vi "Temp Chamber Testing Log w subVIs ver 2.vi"() -> ()   [LabVIEW 2010]
uses:
  <vilib>/Analysis/Matrix/Datatypes/RealMatrix.ctl
  <vilib>/Utility/NIReport.llb/NI_report.lvclass
  <vilib>/Utility/NIReport.llb/Append Numeric Table to Report (wrap).vi
  <vilib>/Utility/NIReport.llb/Excel/NI_Excel.lvclass
  <vilib>/Analysis/Matrix/NI_Matrix.lvlib
panel:
  in  "Wait time (row 1) [mins] and iterations for that time (row 2)":T1
  out "error out":errorcluster
  in  "error in (no error)":errorcluster
  in  "Fiber Len (m)":dbl
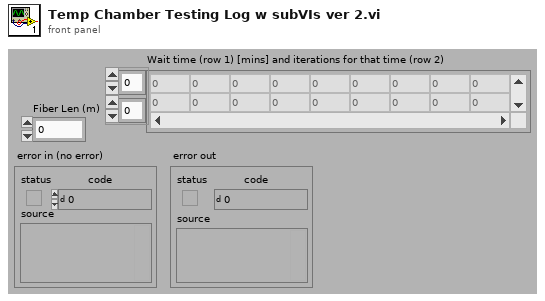
[diagram p1: front panel]
types:
  T1 = typedef "NI_Matrix.lvlib/RealMatrix.ctl" = dbl[][]
  T2 = enum16{"Standard Report", "HTML", "Word", "Excel"}
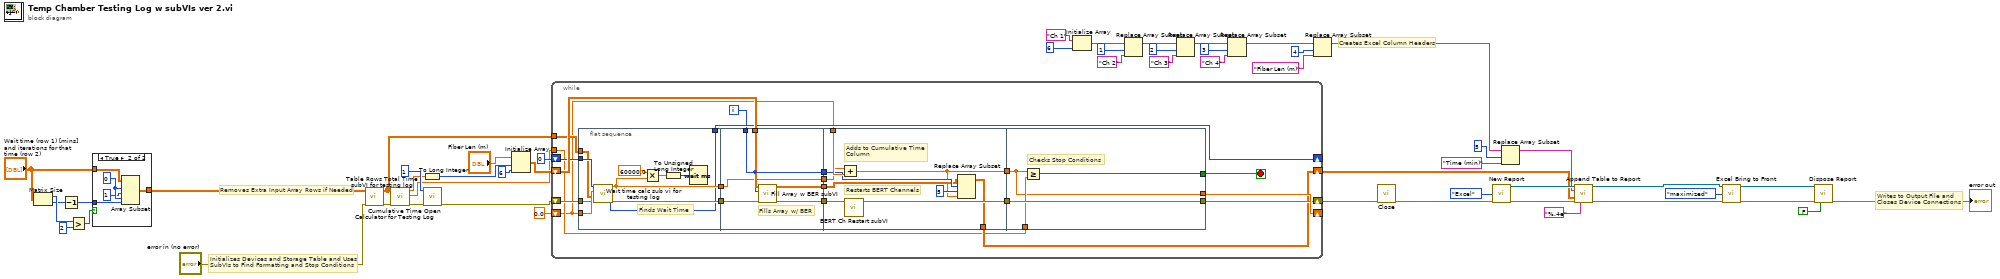
[diagram p0: block diagram]
diagram:
  # "Creates Excel Column Headers"
  # "Removes Extra Input Array Rows if Needed"
  # "Writes to Output File and \nCloses Device Connections"
  # "Initializes Devices and Storage Table and Uses\nSubVIs to Find Formatting and Stop Conditions"
  n1 = Matrix Size(0:"Wait time (row 1) [mins] and iterations for that time (row 2)") -> (1:w26:i32, 2:w22:i32)
  n2 = Decrement(x=w22) -> (x-1=w21:i32)
  n3 = Greater?(x=w26, y=2) -> (0:w24:bool)
  n4 = case shown="True" w24 {
    tunnel: "Wait time (row 1) [mins] and iterations for that time (row 2)" -> [w54 w59]
    tunnel: [w54 w58] -> w20
    tunnel: w21 -> [_ w55]
    frame False {
    }
    frame True {
      w57 = 0
      n5 = Array Subset(array=w59, index (row)=w57, length (row)=1, index (col)=w57, length (col)=w55) -> (w58:T1)
    }
  }
  n6 = call "Cumulative Time Calculator for Testing Log.vi"("error in (no error)"="error in (no error)", "Input Matrix"=w20) -> ("error out"=w27:errorcluster, "Output Matrix"=w29:T1)  [unwired: 8 in]
  n7 = call "Table Rows Total Time subVI for testing log.vi"("error in (no error)"=w27, "Input Matrix"=w29) -> ("error out"=w33:errorcluster, "Total Time (mins)"=w30:dbl, "# of Table Rows"=w32:dbl)  [unwired: 7 in]
  n8 = To Long Integer(number=w32) -> (32bit integer=w31:i32)
  n9 = call <instrlib>:"Open.vi"("error in (no error)"=w33, "type"=1) -> ("error out"=w50:errorcluster)  [unwired: 8 in, 1 out]
  n10 = Initialize Array("Fiber Len (m)", w31, 6) -> (w51:dbl[][])
  n11 = while {
    shift-right: [w65] -> w38
    shift-left: w51 -> [w79]
    shift-right: [w70] -> w35
    shift-left: w50 -> [w77]
    shift-right: [w75] -> _
    shift-left: 0.0 -> [w62]
    shift-right: [w73] -> _
    shift-left: 0 -> [w74]
    tunnel: w29 -> [w64]
    tunnel: w30 -> [w63]
    i -> [w71]
    stop <- w67 stop-if-true
    n12 = flat-sequence {
      tunnel: w77 -> [w86]
      tunnel: [w85] -> w76
      tunnel: w62 -> [w89]
      tunnel: w74 -> [w88]
      tunnel: [w84] -> w73
      tunnel: [w87] -> w72
      tunnel: w64 -> [w83]
      tunnel: w79 -> [w95]
      tunnel: w71 -> [w90]
      tunnel: [w91] -> w78
      tunnel: w76 -> [w92]
      tunnel: w72 -> [w93]
      tunnel: [w94] -> w66
      tunnel: [w93] -> w61
      tunnel: [w90] -> w60
      tunnel: w78 -> [w103]
      tunnel: w62 -> [w104]
      tunnel: [w96] -> w69
      tunnel: [w102] -> w68
      tunnel: w66 -> [w98]
      tunnel: [w97] -> w65
      tunnel: w61 -> [w101]
      tunnel: w60 -> [w99]
      tunnel: [w108] -> w70
      tunnel: [w105] -> w75
      tunnel: w69 -> [w105]
      tunnel: w68 -> [w108]
      tunnel: [w107] -> w67
      tunnel: w63 -> [w106]
      frame #0 {
        # "Finds Wait Time"
        n13 = call "Wait time calc sub vi for testing log.vi"("error in (no error)"=w86, "Input matrix"=w83, "Elapsed time (min)"=w89, "Input column"=w88) -> ("error out"=w85:errorcluster, "Column out"=w84:i32, "Wait time (min)"=w87:dbl)  [unwired: 5 in]
        n14 = Multiply(x=60000.0, y=w87) -> (x*y=w81:dbl)
        n15 = To Unsigned Long Integer(number=w81) -> (unsigned 32bit integer=w80:u32)
        n16 = Wait (ms)(milliseconds to wait=w80) -> ()  [unwired: 1 out]
      }
      frame #1 {
        # "Fills Array w/ BER"
        n17 = call "Fill Array w BER subVI.vi"("error in (no error)"=w92, "Index"=w90, "Building Array In"=w95) -> ("error out"=w91:errorcluster, "Building Array Out"=w94:dbl[][])  [unwired: 7 in]
      }
      frame #2 {
        # "Adds to Cumulative Time\nColumn"
        # "Restarts BERT Channels"
        n18 = Add(x=w101, y=w104) -> (x+y=w96:dbl)
        n19 = call "BERT Ch Restart subVI.vi"("error in (no error)"=w103) -> ("error out"=w102:errorcluster)  [unwired: 10 in]
        n20 = Replace Array Subset(array=w98, new element=w96, index (row)=w99, index (col)=5) -> (w97:dbl[][])
      }
      frame #3 {
        # "Checks Stop Conditions"
        n21 = Greater Or Equal?(x=w105, y=w106) -> (x >= y?=w107:bool)
      }
    }
  }
  n22 = Initialize Array("Ch 1", 6) -> (w17:string[])
  n23 = Replace Array Subset(array=w17, new element="Ch 2", index=1) -> (w15:string[])
  n24 = Replace Array Subset(array=w15, new element="Ch 3", index=2) -> (w13:string[])
  n25 = Replace Array Subset(array=w13, new element="Ch 4", index=3) -> (w10:string[])
  n26 = Replace Array Subset(array=w10, new element="Fiber Len (m)", index=4) -> (w9:string[])
  n27 = call <instrlib>:"Close.vi"("error in (no error)"=w35) -> ("error out"=w40:errorcluster)  [unwired: 9 in, 1 out]
  n28 = call <vilib>:"New Report.vi"("report type"=T2."Excel", "error in (no error)"=w40) -> ("report out"=w48:refnum<class "NI_report.lvclass">, "error out"=w47:errorcluster)  [unwired: 4 in, 8 out]
  n29 = Replace Array Subset(array=w9, new element="Time (min)", index=5) -> (w2:string[])
  n30 = call-poly <vilib>:"Append Table to Report.vi"("report in"=w48, "column headers"=w2, "numerical data"=w38, "error in (no error)"=w47, "format string (%.3f)"="%.4e") -> ("report out"=w45:refnum<class "NI_report.lvclass">, "error out"=w44:errorcluster)  [unwired: 5 in, 4 out]
  n31 = call <vilib>:"Excel Bring to Front.vi"("report in"=w45, "window state (maximized)"=enum16{"maximized", "minimized", "normal"}."maximized", "error in (no error)"=w44) -> ("report out"=w42:refnum<class "NI_report.lvclass">, "error out"=w43:errorcluster)  [unwired: 11 out]
  n32 = call-dynamic "Dispose Report.vi"("report in"=w42, "error in (no error)"=w43, "close report? (T)"=FALSE) -> ("error out"=→"error out":errorcluster)  [unwired: 2 in, 10 out]
